vi "MotorMain.vi"(8 "SetPosition waittime (30)":u32=30) -> ()   [LabVIEW 2011]
uses:
  Modules/PIMotorController/PI_Axis_list.ctl
  Modules/PIMotorController/PI_Axis.ctl
  Main/Motors/MotorConfigType.ctl
  Main/Motors/MotorPosType.ctl
  Main/Typedefs/XYf.ctl
  Main/Motors/MotorPosFlagsType.ctl
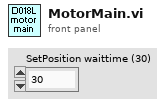
[diagram p1: front panel]
types:
  T1 = typedef "PI_Axis_list.ctl" = cluster{"Piezo X":T2, "Piezo Y":T2, "Piezo Z":T2, "Magnet Z":T2, "Magnet Rotation":T2, "Objective X":T2, "Objective Y":T2}
  T2 = typedef "PI_Axis.ctl" = cluster{"System #":i32, "Axis ID":string, "Multiplier":dbl}
  T3 = typedef "MotorConfigType.ctl" = cluster{"Offset":T4, "Maximum pos":T4, "Min limited?":T6, "Max limited?":T6, "Has velocity support":T6, "Default velocity":T4}
  T4 = typedef "MotorPosType.ctl" = cluster{"Magnet Z":dbl, "Magnet rotation":dbl, "Camera":T5, "Piezo XY":T5, "Piezo Z":dbl}
  T5 = typedef "XYf.ctl" = cluster{"X":sgl, "Y":sgl}
  T6 = typedef "MotorPosFlagsType.ctl" = cluster{"Magnet Z":bool, "Magnet rotation":bool, "Camera":cluster{"X":bool, "Y":bool}, "Piezo XY":cluster{"X":bool, "Y":bool}, "Piezo Z":bool}
  T7 = typedef "GCS_Interface.ctl" = cluster{"MOV":refnum<vi>, "VEL":refnum<vi>, "VEL?":refnum<vi>, "POS?":refnum<vi>, "TMX?":refnum<vi>, "#7 (Ready?)":refnum<vi>, "FPL":refnum<vi>, "FNL":refnum<vi>}
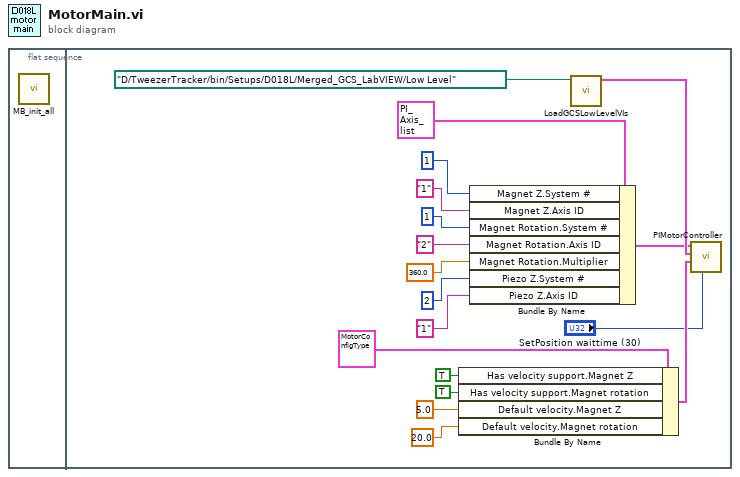
[diagram p0: block diagram]
diagram:
  n1 = flat-sequence {
    frame #0 {
      n2 = call "MB_init_all.vi"() -> ()  [unwired: 12 in]
    }
    frame #1 {
      n3 = Bundle By Name(cluster=T3 {"Offset"={"Magnet Z"=0.0, "Magnet rotation"=0.0, "Camera"={"X"=0.0, "Y"=0.0}, "Piezo XY"={"X"=0.0, "Y"=0.0}, "Piezo Z"=0.0}, "Maximum pos"={"Magnet Z"=0.0, "Magnet rotation"=0.0, "Camera"={"X"=0.0, "Y"=0.0}, "Piezo XY"={"X"=0.0, "Y"=0.0}, "Piezo Z"=0.0}, "Min limited?"={"Magnet Z"=FALSE, "Magnet rotation"=FALSE, "Camera"={"X"=FALSE, "Y"=FALSE}, "Piezo XY"={"X"=FALSE, "Y"=FALSE}, "Piezo Z"=FALSE}, "Max limited?"={"Magnet Z"=FALSE, "Magnet rotation"=FALSE, "Camera"={"X"=FALSE, "Y"=FALSE}, "Piezo XY"={"X"=FALSE, "Y"=FALSE}, "Piezo Z"=FALSE}, "Has velocity support"={"Magnet Z"=TRUE, "Magnet rotation"=TRUE, "Camera"={"X"=FALSE, "Y"=FALSE}, "Piezo XY"={"X"=FALSE, "Y"=FALSE}, "Piezo Z"=FALSE}, "Default velocity"={"Magnet Z"=0.0, "Magnet rotation"=0.0, "Camera"={"X"=0.0, "Y"=0.0}, "Piezo XY"={"X"=0.0, "Y"=0.0}, "Piezo Z"=0.0}} ("MotorConfig"), "Has velocity support.Magnet Z"=TRUE, "Has velocity support.Magnet rotation"=TRUE, "Default velocity.Magnet Z"=5.0, "Default velocity.Magnet rotation"=20.0) -> (w15:T3)
      n4 = Bundle By Name(cluster=T1 {"Piezo X"={"System #"=0, "Axis ID"="", "Multiplier"=1.0}, "Piezo Y"={"System #"=0, "Axis ID"="", "Multiplier"=1.0}, "Piezo Z"={"System #"=0, "Axis ID"="", "Multiplier"=1.0}, "Magnet Z"={"System #"=0, "Axis ID"="", "Multiplier"=1.0}, "Magnet Rotation"={"System #"=0, "Axis ID"="", "Multiplier"=1.0}, "Objective X"={"System #"=0, "Axis ID"="", "Multiplier"=1.0}, "Objective Y"={"System #"=0, "Axis ID"="", "Multiplier"=1.0}} ("PI Axis config"), "Magnet Z.System #"=1, "Magnet Z.Axis ID"="1", "Magnet Rotation.System #"=1, "Magnet Rotation.Axis ID"="2", "Magnet Rotation.Multiplier"=360.0, "Piezo Z.System #"=2, "Piezo Z.Axis ID"="1") -> (w11:T1)
      n5 = call "LoadGCSLowLevelVIs.vi"("GCS Merged Drivers Low-Level Path"=path "D:/TweezerTracker/bin/Setups/D018L/Merged_GCS_LabVIEW/Low Level") -> ("PI GCS Function\nReferences"=w18:T7)  [unwired: 10 in]
      n6 = call "PIMotorController.vi"("SetPosition waittime (30)"="SetPosition waittime (30)", "MotorConfig"=w15, "PI GCS Function\nReferences"=w18, "PI Axis config"=w11) -> ()  [unwired: 8 in]
    }
  }
